vi "Channel_mapping.vi"(11 "Channel IN":i32=16) -> (3 "Operating \nChannel(s)":bool[][](array[boolean]))   [LabVIEW 2023]
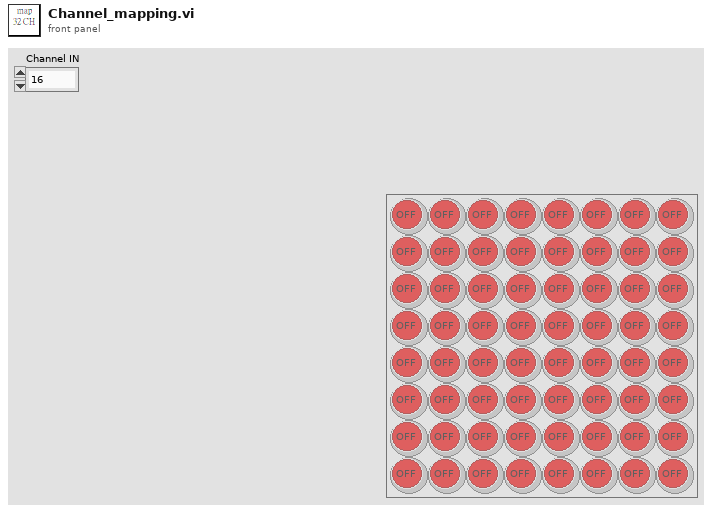
[diagram p1: front panel]
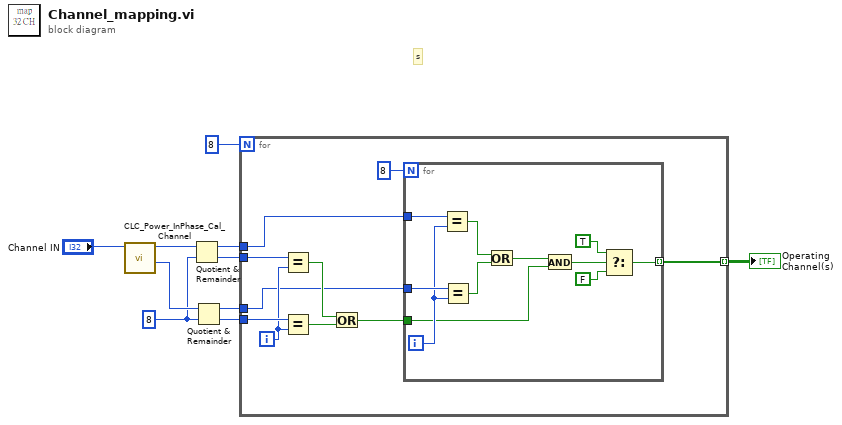
[diagram p0: block diagram]
diagram:
  w4 = 8 ("y")
  # "s"
  n1 = call "CLC_Power_InPhase_Cal_Channel.vi"("Channel IN"="Channel IN") -> ("Channel"=w8:i32, "Ref_Channel"=w5:i32)  [unwired: 8 in, 1 out]
  n2 = Quotient & Remainder(x=w5, y=w4) -> (x-y*floor(x/y)=w3:i32, floor(x/y)=w2:i32)
  n3 = Quotient & Remainder(x=w8, y=w4) -> (x-y*floor(x/y)=w6:i32, floor(x/y)=w7:i32)
  n4 = for {
    N: 8 -> [_]
    tunnel: [w19] -> w9 mode=indexing
    tunnel: w7 -> [w18]
    tunnel: w6 -> [w11]
    tunnel: w3 -> [w12]
    tunnel: w2 -> [w17]
    i -> [w16]
    n5 = Equal?(x=w17, y=w16) -> (x = y?=w14:bool)
    n6 = Equal?(x=w18, y=w16) -> (x = y?=w15:bool)
    n7 = Or(x=w14, y=w15) -> (x .or. y?=w13:bool)
    n8 = for {
      N: 8 -> [_]
      tunnel: [w22] -> w19 mode=indexing
      tunnel: w13 -> [w26]
      tunnel: w12 -> [w31]
      tunnel: w11 -> [w30]
      i -> [w29]
      n9 = Equal?(x=w31, y=w29) -> (x = y?=w28:bool)
      n10 = Equal?(x=w30, y=w29) -> (x = y?=w27:bool)
      n11 = Or(x=w28, y=w27) -> (x .or. y?=w25:bool)
      n12 = And(x=w25, y=w26) -> (x .and. y?=w21:bool)
      n13 = Select(t=TRUE, s=w21, f=FALSE) -> (s? t:f=w22:bool)
    }
  }
  "Operating \nChannel(s)" <- w9
